vi "List Packages.vi"(8 "error in (no error)":errorcluster, 11 "GCentral API in":refnum<class "GCentral API.lvclass">) -> (0 "error out":errorcluster, 2 "Packages":refnum<class "Package.lvclass">[](array[class]), 3 "GCentral API out":refnum<class "GCentral API.lvclass">, 4 "Debug Link":string)   [LabVIEW 2020, in "GCentral-API.lvlib" / "GCentral API.lvclass"]
uses:
  GCentral API.lvclass
  Package/Package.lvclass
  API Endpoint.ctl
  GCentral-API.lvlib
  neg-pkg/JSON/JSON.lvlib
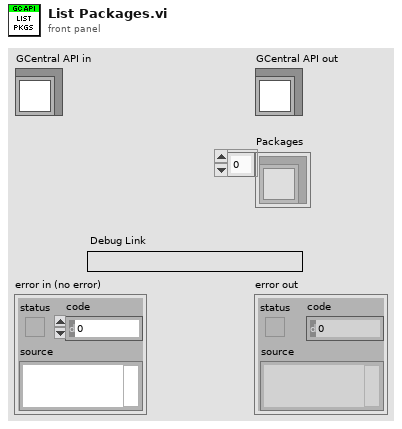
[diagram p1: front panel]
types:
  T1 = typedef "GCentral-API.lvlib/API Endpoint.ctl" = enum16{"packages/list", "packages/search"}
  T2 = typedef "JSON.lvlib/JSON Item Type.ctl" = enum16{"unknown", "null", "Array", "Object", "String", "Number", "Boolean"}
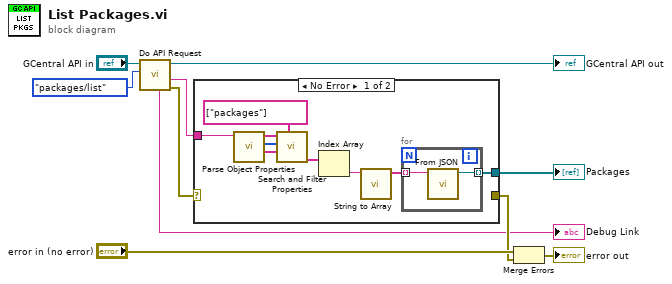
[diagram p0: block diagram]
diagram:
  n1 = call "Do API Request.vi"("API Endpoint"=API_Endpoint."packages/list", "GCentral API in"="GCentral API in") -> ("error out"=w5:errorcluster, "Response"=w6:string, "GCentral API out"=→"GCentral API out":refnum<class "GCentral API.lvclass">, "Debug Link"=→"Debug Link":string)  [unwired: 5 in, 1 out]
  n2 = case shown="No Error" w5 {
    selector: w5 -> [_ w22]
    tunnel: w6 -> [w13 _]
    tunnel: [w11 _] -> w9
    tunnel: [_ w22] -> w7
    frame No Error {
      n3 = call "Parse Object Properties.vi"("JSON String"=w13) -> ("Values"=w17:string[], "Item Types"=w18:T2[], "Keys"=w19:string[])  [unwired: 7 in, 1 out]
      n4 = call "Search and Filter Properties.vi"("Search Keys"=string[] ["packages"], "Values In"=w17, "Types In"=w18, "Keys In"=w19) -> ("Filtered Values"=w15:string[])  [unwired: 2 in, 5 out]
      n5 = Index Array(array=w15) -> (element=w14:string)  [unwired: 1 in]
      n6 = call "String to Array.vi"("Array String In"=w14) -> ("JSON Strings"=w12:string[])  [unwired: 10 in]
      n7 = for {
        tunnel: w12 -> [w21] mode=indexing
        tunnel: [w20] -> w11 mode=indexing
        n8 = call "From JSON.vi"("JSON"=w21) -> ("Package out"=w20:refnum<class "Package.lvclass">)  [unwired: 9 in, 1 out]
      }
    }
    frame Error {
    }
  }
  "Packages" <- w9
  n9 = Merge Errors("error in (no error)", w7) -> (→"error out":errorcluster)
